vi "Set Command To String.vi"(10 "Arguments":variant, 11 "Command":string) -> (3 "data string":string)   [LabVIEW 2017, in "Message Interface.lvlib" / "Command.lvclass"]
uses:
  Command.lvclass
  C:/Users/Public/Documents/wc/BuildFarm/src/LabVIEW/vi.lib/BenjaminR/Build Farm/Classes/Message Interface/iMessage/iMessage.lvclass
  Command.lvclass/Command.ctl
  iMessage/iMessage.lvclass
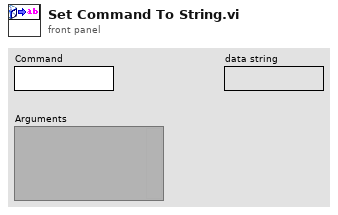
[diagram p1: front panel]
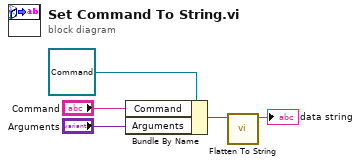
[diagram p0: block diagram]
diagram:
  n1 = Bundle By Name(cluster=refnum<class "Command.lvclass"> refnum ("Command.lvclass"), "Command"="Command", "Arguments"="Arguments") -> (w2:refnum<class "Command.lvclass">)
  n2 = call "Flatten To String.vi"("iMessage in"=w2) -> ("data string"=→"data string":string)  [unwired: 9 in, 1 out]
